vi "Map.vi"(7 "Action":enum8{"noop", "get", "set", "pop"}(ring), 10 "Timer in":T1, 11 "Timer Id":cluster{"Queue":refnum<queue>, "Message":string}) -> (1 "Found?":bool, 2 "Timer out":T1)   [LabVIEW 2018, in "QueueTimer.lvlib"]
doc: "Queue timer in memory cache. Queue timers are identified by `<queue>+<timer_message>`.\n\nNote: Timer messages must be unique."
uses:
  QueueTimer.lvlib
  TypeDefs/Timer.ctl
panel:
  # "Missing object. The object \"Map\" does not exist in the previous version."
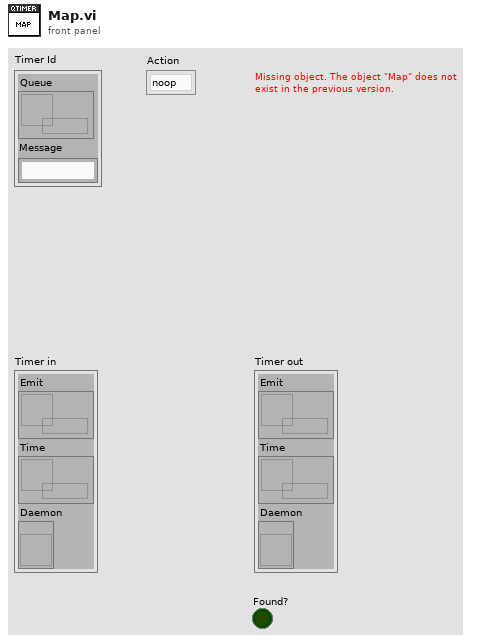
[diagram p1: front panel]
types:
  T1 = cluster{"Emit":refnum<queue>, "Time":refnum<data-value>, "Daemon":refnum<vi>}
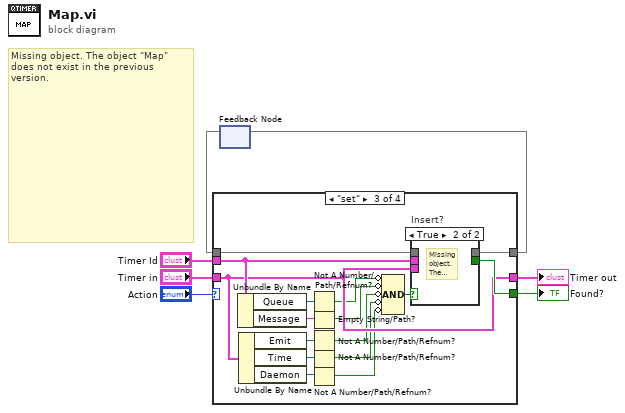
[diagram p0: block diagram]
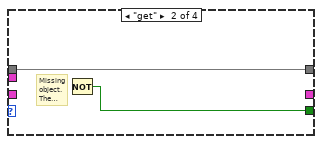
[diagram p3: hidden frame]
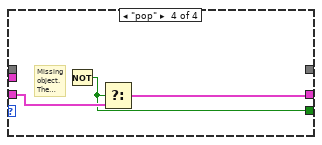
[diagram p5: hidden frame]
diagram:
  # "Missing object. The object \"Map\" does not exist in the previous version."
  n1 = feedback #1() -> (w5, w7)
  n2 = case shown="\"set\"" "Action" {
    tunnel: [w9 w12 w24 w32] -> w8
    tunnel: "Timer Id" -> [_ _ w25 _]
    tunnel: w5 -> [w10 w13 w29 _]
    tunnel: [w10 w13 w28 w35] -> w4
    tunnel: [_ w11 w26 w31] -> w3
    tunnel: "Timer in" -> [w9 _ w24 w34]
    frame "noop" {
    }
    frame "get" {
      # "Missing object. The object \"Look In Map\" does not exist in the previous version."
      n3 = Not() -> (.not. x?=w11:bool)  [unwired: 1 in]
    }
    frame "set" {
      n4 = Unbundle By Name(w25) -> ("Queue"=w21:refnum<queue>, "Message"=w20:string)
      n5 = Unbundle By Name(w24) -> ("Emit"=w23:refnum<queue>, "Time"=w22:refnum<data-value>, "Daemon"=w15:refnum<vi>)
      n6 = Not A Number/Path/Refnum?(number/path/refnum=w21) -> (NaN/Path/Refnum?=w19:bool)
      n7 = Empty String/Path?(string/path=w20) -> (empty?=w18:bool)
      n8 = Not A Number/Path/Refnum?(number/path/refnum=w23) -> (NaN/Path/Refnum?=w17:bool)
      n9 = Not A Number/Path/Refnum?(number/path/refnum=w22) -> (NaN/Path/Refnum?=w16:bool)
      n10 = Not A Number/Path/Refnum?(number/path/refnum=w15) -> (NaN/Path/Refnum?=w14:bool)
      n11 = Compound Arithmetic op=AND(invert w19, invert w18, invert w17, invert w16, invert w14) -> (w27:bool)
      n12 = case "Insert?" shown="True" w27 {
        tunnel: w29 -> [w30 _]
        tunnel: w24 -> [_ _]
        tunnel: w25 -> [_ _]
        tunnel: [w30 _] -> w28
        tunnel: [_ _] -> w26
        frame False {
        }
        frame True {
          # "Missing object. The object \"Insert Into Map\" does not exist in the previous version."
        }
      }
    }
    frame "pop" {
      # "Missing object. The object \"Remove From Map\" does not exist in the previous version."
      n13 = Not() -> (.not. x?=w31:bool)  [unwired: 1 in]
      n14 = Select(s=w31, f=w34) -> (t=w33:T1, s? t:f=w32:T1)
    }
  }
  "Timer out" <- w8
  "Found?" <- w3
  n15 = feedback-in #1(w4) -> ()
